vi "XY Graph Graph Axes Chooser Dialog.vi"(8 "Error In":errorcluster, 11 "XYGraph Ref":refnum<vi>) -> (0 "Error Out":errorcluster, 1 "Message":string, 2 "Cancelled":bool, 3 "XYGraph Ref dup":refnum<vi>)   [LabVIEW 2021, in "XY Graph Add-Ons.lvlib"]
uses:
  XY Graph Add-Ons.lvlib
panel:
  out "Y Scale":i32
  out "X Scale":i32
  in  "Y Axes":i32(listbox)
  in  "X Axes":i32(listbox)
  in  "Cancel":bool
  in  "OK":bool
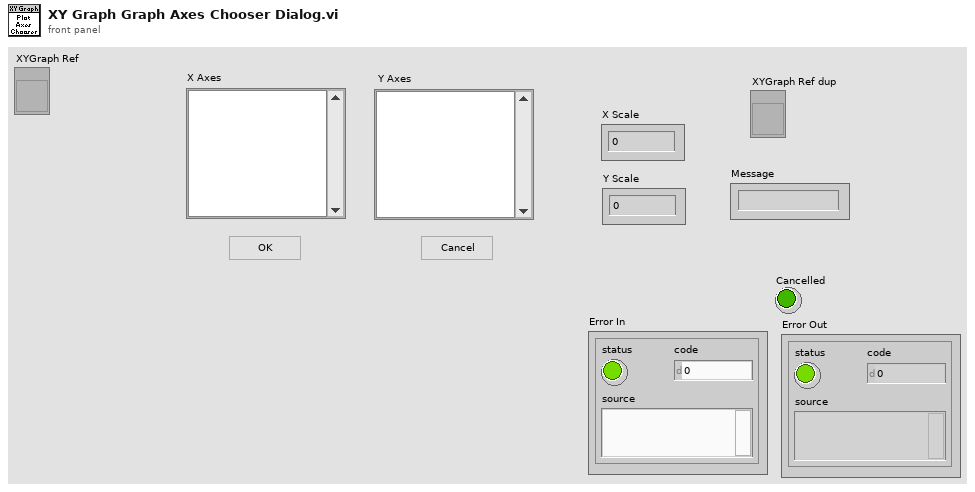
[diagram p1: front panel]
types:
  T1 = typedef "XY Graph Add-Ons.lvlib/XY Graph Refnum.ctl" = refnum<vi>
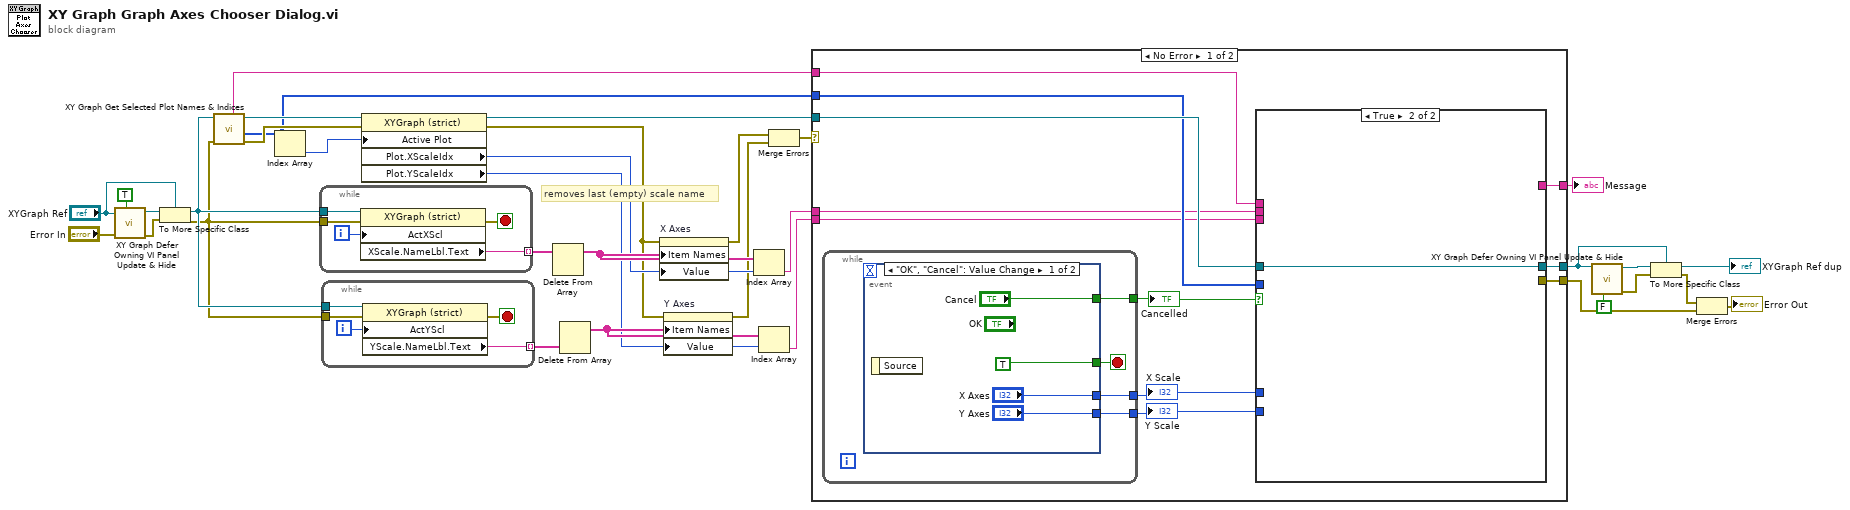
[diagram p0: block diagram]
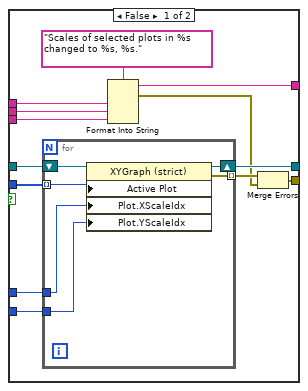
[diagram p2: hidden frame]
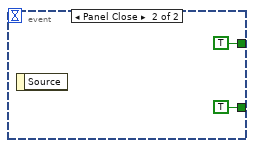
[diagram p3: hidden frame]
diagram:
  # "removes last (empty) scale name"
  n1 = call "XY Graph Defer Owning VI Panel Update & Hide.vi"("Defer Owning Panel Update"=TRUE, "error in (no error)"="Error In", "XY Graph Refnum in"="XYGraph Ref") -> ("error out"=w18:errorcluster, "XY Graph Refnum out"=w16:refnum<vi>)  [unwired: 7 in]
  n2 = To More Specific Class(target class="XYGraph Ref", reference=w16, error in=w18) -> (specific class reference=w14:refnum<vi>, error out=w13:errorcluster)
  n3 = call "XY Graph Get Selected Plot Names & Indices.vi"("error in (no error)"=w13, "XYGraph in"=w14) -> ("error out"=w31:errorcluster, "Selected Plots"=w28:i32[], "XYGraph out"=w32:T1, "Graph Name"=w27:string)  [unwired: 5 in, 1 out]
  n4 = Index Array(array=w28) -> (element=w30:i32)  [unwired: 1 in]
  n5 = while {
    tunnel: w14 -> [w39]
    tunnel: [w36] -> w34 mode=indexing
    tunnel: w13 -> [w35]
    i -> [w38]
    stop <- w37 stop-if-true
    n6 = property class="XYGraph (strict)"(reference=w39, error in=w35, "ActXScl"=w38) -> (error out=w37:errorcluster, "XScale.NameLbl.Text"=w36:string)  [unwired: 1 out]
  }
  n7 = while {
    tunnel: w14 -> [w44]
    tunnel: [w41] -> w33 mode=indexing
    tunnel: w13 -> [w40]
    i -> [w43]
    stop <- w42 stop-if-true
    n8 = property class="XYGraph (strict)"(reference=w44, error in=w40, "ActYScl"=w43) -> (error out=w42:errorcluster, "YScale.NameLbl.Text"=w41:string)  [unwired: 1 out]
  }
  n9 = property class="XYGraph (strict)"(reference=w32, error in=w31, "Active Plot"=w30) -> (reference out=w29:T1, error out=w7:errorcluster, "Plot.XScaleIdx"=w24:u32, "Plot.YScaleIdx"=w22:u32)
  n10 = Delete From Array(array=w34) -> (array with subset deleted=w25:string[])  [unwired: 2 in, 1 out]
  n11 = Delete From Array(array=w33) -> (array with subset deleted=w23:string[])  [unwired: 2 in, 1 out]
  n12 = property on="X Axes" class="LstBox (strict)"(error in=w7, "Item Names"=w25, "Value"=w24) -> (error out=w6:errorcluster)  [unwired: 1 in, 1 out]
  n13 = property on="Y Axes" class="LstBox (strict)"(error in=w7, "Item Names"=w23, "Value"=w22) -> (error out=w5:errorcluster)  [unwired: 1 in, 1 out]
  n14 = Index Array(array=w25, index=w24) -> (element=w21:string)
  n15 = Index Array(array=w23, index=w22) -> (element=w20:string)
  n16 = Merge Errors(w6, w5) -> (w4:errorcluster)
  n17 = case shown="No Error" w4 {
    selector: w4 -> [_ w86]
    tunnel: w29 -> [w54 w87]
    tunnel: w28 -> [w53 _]
    tunnel: w27 -> [w50 _]
    tunnel: [w49 _] -> w26
    tunnel: w21 -> [w48 _]
    tunnel: w20 -> [w47 _]
    tunnel: [w46 w87] -> w12
    tunnel: [w45 w86] -> w1
    frame No Error {
      n18 = while {
        tunnel: [w78] -> w55
        tunnel: [w77] -> w52
        tunnel: [w76] -> w51
        stop <- w79 stop-if-true
        n19 = event shown="[0] \"OK\", \"Cancel\": Value Change" {
          selector: _ -> [_ _]
          dyn-events: _ -> [_ _]
          timeout: _ -> [_ _]
          tunnel: [TRUE TRUE] -> w79
          tunnel: ["Cancel" TRUE ("Cancel")] -> w78
          tunnel: ["X Axes" _] -> w77
          tunnel: ["Y Axes" _] -> w76
          event "OK", "Cancel": Value Change {
            n20 = event-data() -> ()  [unwired: 1 in, 1 out]
          }
          event Panel Close {
            n21 = event-data() -> ()  [unwired: 1 in, 1 out]
          }
        }
      }
      "Cancelled" <- w55
      "X Scale" <- w52
      "Y Scale" <- w51
      n22 = case shown="True" w55 {
        tunnel: w54 -> [w68 w75]
        tunnel: w53 -> [w67 _]
        tunnel: w52 -> [w66 _]
        tunnel: w51 -> [w65 _]
        tunnel: w50 -> [w64 _]
        tunnel: [w62 _] -> w49
        tunnel: w48 -> [w61 _]
        tunnel: w47 -> [w60 _]
        tunnel: [w59 w75] -> w46
        tunnel: [w56 _] -> w45
        frame False {
          n23 = for {
            tunnel: w67 -> [w73] mode=indexing
            tunnel: w66 -> [w72]
            tunnel: w65 -> [w71]
            shift-right: [w70] -> w59
            shift-left: w68 -> [w74]
            tunnel: [w69] -> w58 mode=indexing
            n24 = property class="XYGraph (strict)"(reference=w74, "Active Plot"=w73, "Plot.XScaleIdx"=w72, "Plot.YScaleIdx"=w71) -> (reference out=w70:T1, error out=w69:errorcluster)  [unwired: 1 in]
          }
          n25 = Format Into String(format string="Scales of selected plots in %s changed to %s, %s.", w64, w61, w60) -> (resulting string=w62:string, error out=w57:errorcluster)  [unwired: 2 in]
          n26 = Merge Errors(w58, w57) -> (w56:errorcluster)
        }
        frame True {
        }
      }
    }
    frame Error {
    }
  }
  "Message" <- w26
  n27 = call "XY Graph Defer Owning VI Panel Update & Hide.vi"("Defer Owning Panel Update"=FALSE, "XY Graph Refnum in"=w12) -> ("error out"=w10:errorcluster, "XY Graph Refnum out"=w11:refnum<vi>)  [unwired: 8 in]
  n28 = To More Specific Class(target class=w12, reference=w11, error in=w10) -> (specific class reference=→"XYGraph Ref dup":T1, error out=w9:errorcluster)
  n29 = Merge Errors(w9, w1) -> (→"Error Out":errorcluster)
